vi "replace string subset in binary file.vi"(3 "error in":errorcluster, 5 "file path (use dialog)":path) -> (0 "error out":errorcluster)   [LabVIEW 2013]
panel:
  out "length 3":i32
  out "length 2":i32
  out "length":i32
  out "data 2":string
  out "result string":string
  out "offset past replacement":i32
  out "number of replacements":i32
  out "data":string
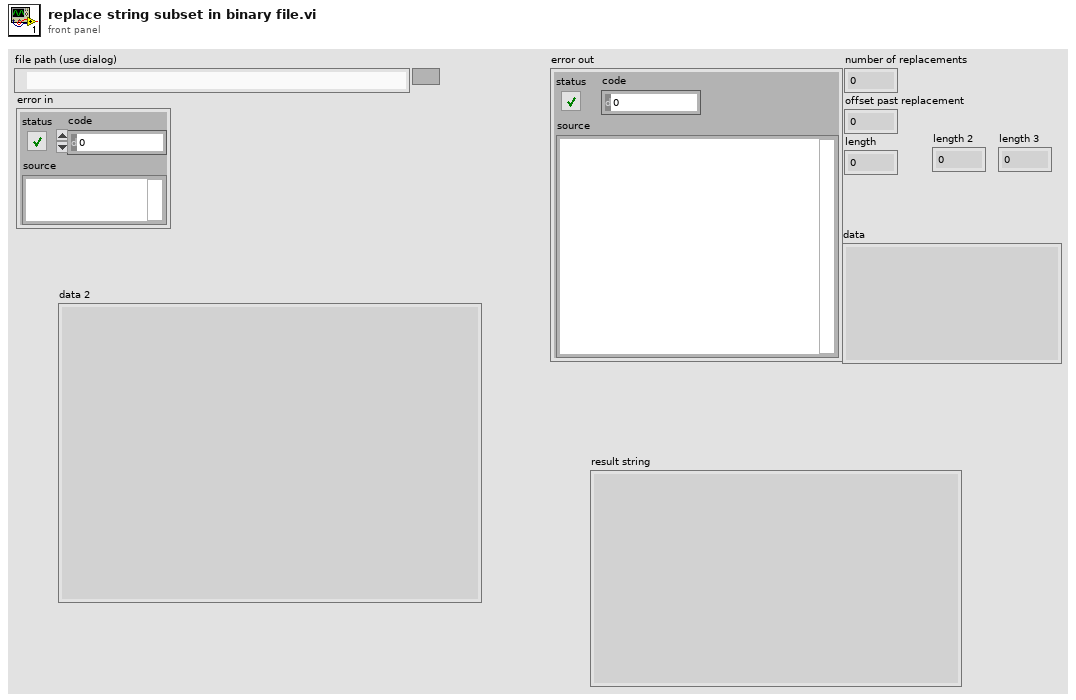
[diagram p1: front panel]
types:
  T1 = enum16{"open", "replace", "create", "open or create", "replace or create", "replace or create with confirmation"}
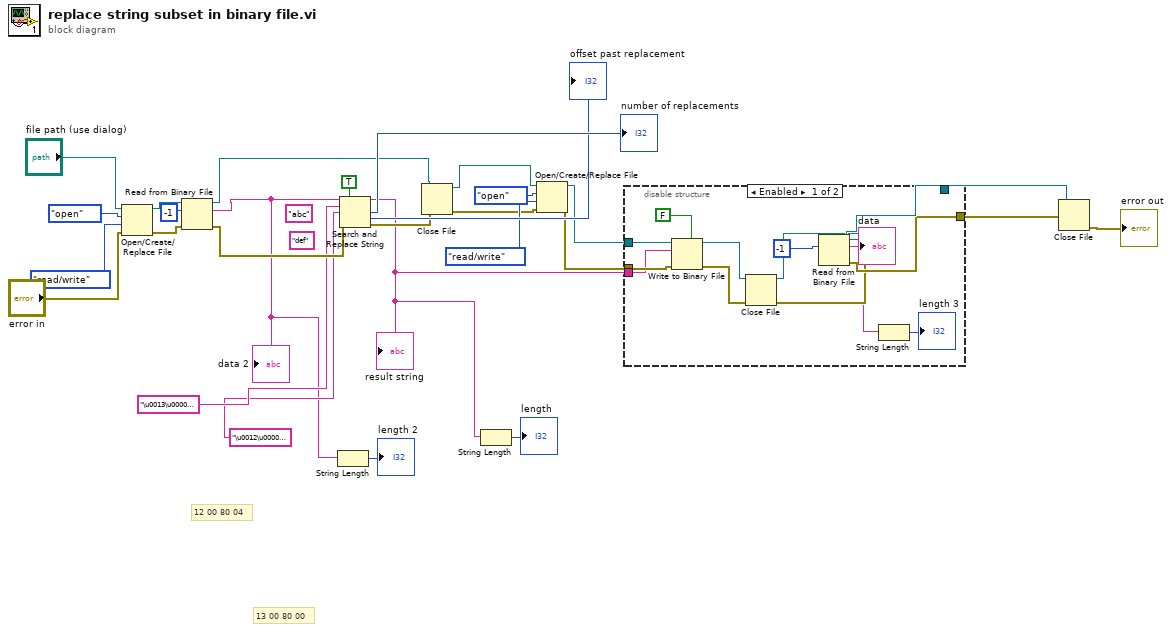
[diagram p0: block diagram]
diagram:
  (unwired) "def" ("search string")
  (unwired) "abc" ("search string")
  # "13 00 80 00"
  # "12 00 80 04"
  n1 = Open/Create/Replace File(file path (use dialog)="file path (use dialog)", error in="error in", operation (0:open)=T1."open", access (0:read/write)=enum16{"read/write", "read-only", "write-only"}."read/write") -> (refnum out=w22:refnum<file>, error out=w21:errorcluster)  [unwired: 2 in, 1 out]
  n2 = Read from Binary File(8:w21, 10:-1 ("count (1)"), 11:w22) -> (0:w16:errorcluster, 2:w1:string, 3:w15:refnum<file>)  [unwired: 3 in, 1 out]
  "data 2" <- w1
  n3 = String Length(string=w1) -> (length=→"length 2":i32)
  n4 = Search and Replace String(replace all?=TRUE ("replace all? (F)"), input string=w1, search string="\u0013\u0000€\u0000", replace string="\u0012\u0000€\u0004" ("search string"), error in=w16) -> (result string=w4:string, number of replacements=→"number of replacements":i32, offset past replacement=→"offset past replacement":i32, error out=w14:errorcluster)  [unwired: 3 in]
  "result string" <- w4
  n5 = Close File(refnum=w15, error in=w14) -> (path=w7:path, error out=w10:errorcluster)
  n6 = String Length(string=w4) -> (length=→"length":i32)
  n7 = Open/Create/Replace File(file path (use dialog)=w7, error in=w10, operation (0:open)=T1."open", access (0:read/write)=enum16{"read/write", "read-only", "write-only"}."read/write") -> (refnum out=w9:refnum<file>, error out=w8:errorcluster)  [unwired: 2 in, 1 out]
  n8 = disable-structure shown="Enabled" {
    disable-tunnel: [w40 w43] -> w27
    disable-tunnel: [w39 w42] -> w26
    disable-tunnel: w9 -> [w38 w43]
    disable-tunnel: w8 -> [w37 w42]
    disable-tunnel: w4 -> [w36 _]
    frame Enabled {
      n9 = Write to Binary File(file (use dialog)=w38, data=w36, error in=w37, 5:FALSE ("prepend array or string size? (T)")) -> (refnum out=w35:refnum<file>, error out=w34:errorcluster)  [unwired: 2 in, 1 out]
      n10 = Close File(refnum=w35, error in=w34) -> (path=w32:path, error out=w33:errorcluster)
      n11 = Read from Binary File(8:w33, 10:-1 ("count (1)"), 11:w32) -> (0:w39:errorcluster, 2:w29:string, 3:w40:refnum<file>)  [unwired: 3 in, 1 out]
      "data" <- w29
      n12 = String Length(string=w29) -> (length=→"length 3":i32)
    }
    frame Disabled {
    }
  }
  n13 = Close File(refnum=w27, error in=w26) -> (error out=→"error out":errorcluster)  [unwired: 1 out]
